vi "Display Frequencies.vi"() -> ()   [LabVIEW 8.6]
uses:
  <vilib>/measure/NI_MABase.lvlib
  <vilib>/express/express analysis/Spectral/XNode/ExpressSpectralMeasurementsBlockNode.xnode
  <vilib>/measure/NI_MAPro.lvlib
  <vilib>/measure/mamon.llb/Waveform Peak Detection for 1 Chan.vi
  <vilib>/express/express analysis/Spectral/Block/exnSpectralBlock spectral measurements RMS poly.vi
  <vilib>/express/express analysis/Spectral/Block/exnSpectralBlock spectral measurements RMS array WFM.vi
panel:
  out "FFT Signal":cluster{"f0":dbl, "df":dbl, "magnitude":dbl[]}[](graph)
  out "Frequencies":dbl[][](array[numeric])
  out "Input Signal":dynamicdata(graph)
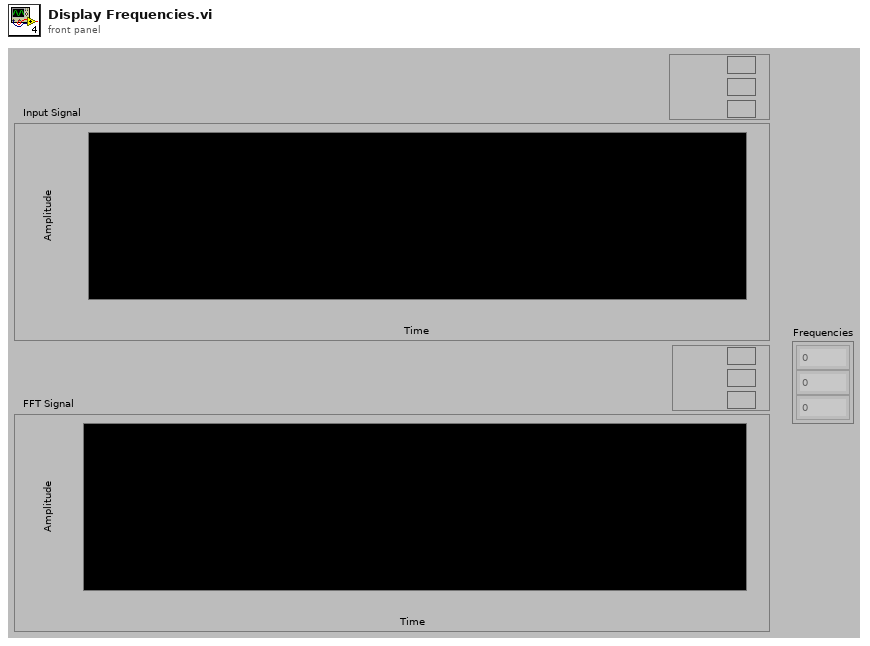
[diagram p1: front panel]
types:
  T1 = enum16{"Sine Wave", "Triangle Wave", "Square Wave", "Sawtooth Wave"}
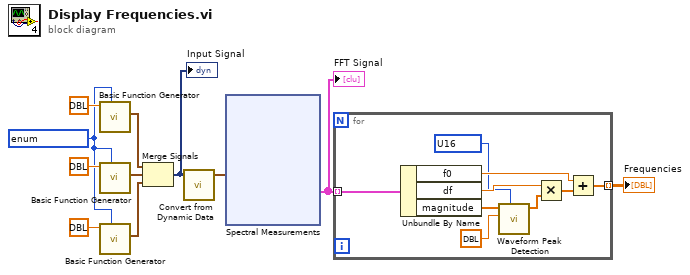
[diagram p0: block diagram]
diagram:
  w8 = T1 ? ("signal type")
  n1 = call <vilib>:"Basic Function Generator.vi"("signal type"=w8, "frequency"=dbl ?) -> ("signal out"=w5:waveform(dbl))  [unwired: 7 in, 2 out]
  n2 = call <vilib>:"Basic Function Generator.vi"("signal type"=w8, "frequency"=dbl ?) -> ("signal out"=w6:waveform(dbl))  [unwired: 7 in, 2 out]
  n3 = call <vilib>:"Basic Function Generator.vi"("signal type"=w8, "frequency"=dbl ?) -> ("signal out"=w7:waveform(dbl))  [unwired: 7 in, 2 out]
  n4 = Merge Signals(w5, w6, w7) -> (w4:dynamicdata)
  "Input Signal" <- w4
  n5 = call "Convert from Dynamic Data"("Dynamic Data Type"=w4) -> ("Array of Waveform"=w3:waveform(dbl)[])  [unwired: 3 in]
  n6 = xnode "Spectral Measurements"("Signals"=w3) -> ("FFT - (RMS)"=w1:cluster{"f0":dbl, "df":dbl, "magnitude":dbl[]}[])  [unwired: 1 in, 2 out]
  "FFT Signal" <- w1
  n7 = for {
    tunnel: w1 -> [w20] mode=indexing
    tunnel: [w12] -> w2 mode=indexing
    w15 = u16 ? items=["Peaks", "Valleys"] ("peaks/valleys")
    n8 = Unbundle By Name(w20) -> ("f0"=w17:dbl, "df"=w16:dbl, "magnitude"=w19:dbl[])
    n9 = call-poly <vilib>:"Waveform Peak Detection.vi"("peaks/valleys"=w15, "threshold"=dbl ?, "Signal In"=w19) -> ("Locations"=w13:dbl[])  [unwired: 4 in, 4 out]
    n10 = Multiply(x=w16, y=w13) -> (x*y=w18:dbl[])
    n11 = Add(x=w17, y=w18) -> (x+y=w12:dbl[])
  }
  "Frequencies" <- w2
